vi "SVN Read Disclaimer.vi"(8 "error in (no error)":errorcluster, 9 "Method version":i32, 10 "Method Name":string) -> (0 "error out":errorcluster, 1 "Valid method":bool, 3 "Disclaimer text":string)   [LabVIEW 2012]
uses:
  ReadWrite.ctl
  Folders.ctl
  Design Server.lvlib
panel:
  out "result string":string
  out "standard error":string
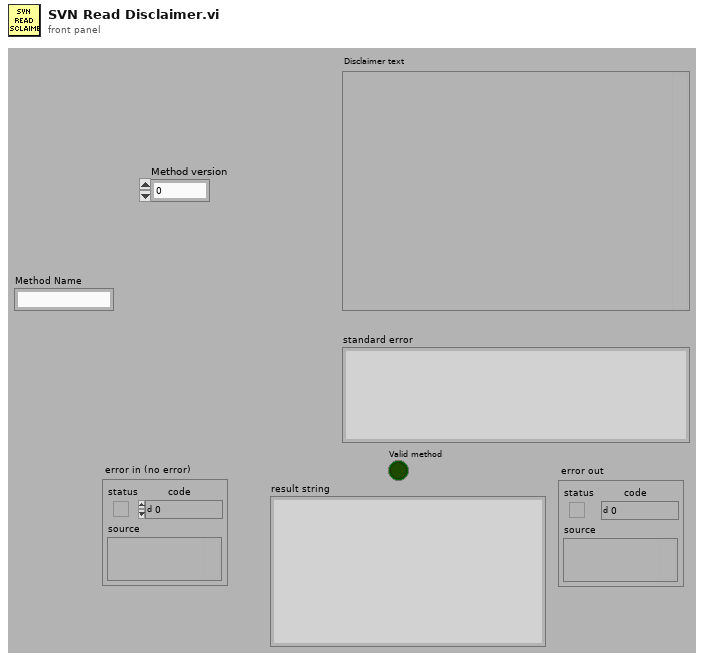
[diagram p1: front panel]
types:
  T1 = typedef "Design Server.lvlib/Folders.ctl" = enum16{"MathcadMethods", "RequestedDesigns", "CompletedDesigns", "MathcadCode", "CollabnetSVN.exe"}
  T2 = typedef "ReadWrite.ctl" = enum16{"Read", "Write"}
  T3 = typedef "SVN.ctl" = cluster{"Mathcad Code Repository":string, "Username":string, "Password":string, "Method file names (w extension)":string}
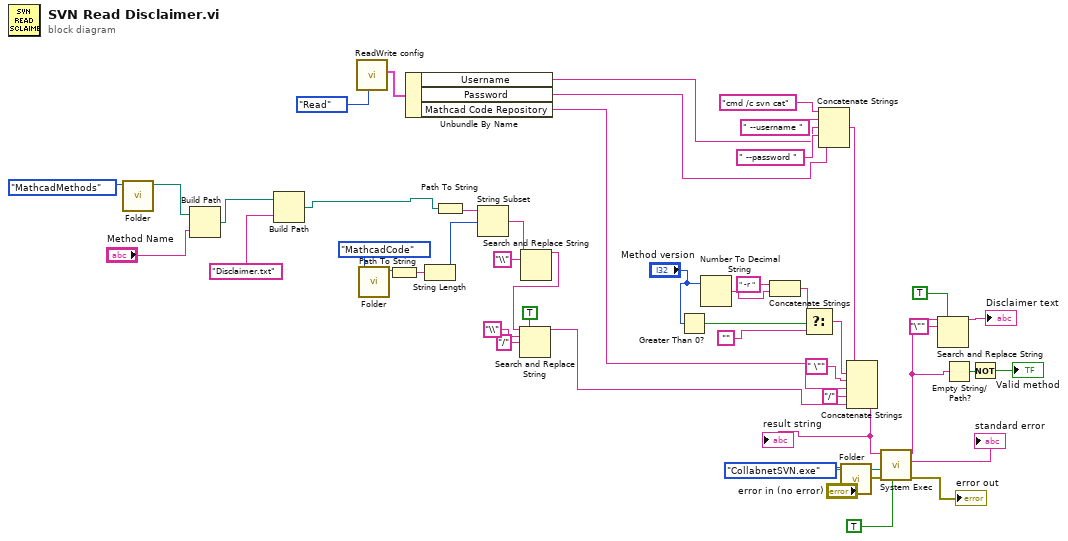
[diagram p0: block diagram]
diagram:
  n1 = call "Folder.vi"("Folders"=Folders."MathcadMethods") -> ("FolderPath"=w4:path)  [unwired: 8 in, 2 out]
  n2 = Build Path(base path=w4, name or relative path="Method Name") -> (appended path=w3:path)
  n3 = Build Path(base path=w3, name or relative path="Disclaimer.txt" ("string")) -> (appended path=w1:path)
  n4 = call "ReadWrite config.vi"("Config"=ReadWrite."Read") -> ("SVN"=w37:T3)  [unwired: 7 in, 3 out]
  n5 = call "Folder.vi"("Folders"=Folders."MathcadCode") -> ("FolderPath"=w25:path)  [unwired: 8 in, 2 out]
  n6 = Path To String(path=w25) -> (string=w26:string)
  n7 = Unbundle By Name(w37) -> ("Username"=w34:string, "Password"=w36:string, "Mathcad Code Repository"=w29:string)
  n8 = String Length(string=w26) -> (length=w22:i32)
  n9 = Path To String(path=w1) -> (string=w2:string)
  n10 = String Subset(string=w2, offset (0)=w22) -> (substring=w21:string)  [unwired: 1 in]
  n11 = Search and Replace String(input string=w21, search string="\\") -> (result string=w18:string)  [unwired: 6 in, 3 out]
  n12 = Search and Replace String(replace all?=TRUE ("replace all? (F)"), input string=w18, search string="\\", replace string="/" ("replace string (\"\")")) -> (result string=w7:string)  [unwired: 4 in, 3 out]
  n13 = Greater Than 0?(x="Method version") -> (x > 0?=w44:bool)
  n14 = Number To Decimal String(number="Method version") -> (decimal integer string=w40:string)  [unwired: 1 in]
  n15 = Concatenate Strings(" -r " ("string"), w40) -> (w42:string)
  n16 = Select(t=w42, s=w44, f="") -> (s? t:f=w39:string)
  n17 = Concatenate Strings("cmd /c svn cat" ("command"), " --username " ("string"), w34, " --password " ("string"), w36) -> (w30:string)
  n18 = call "Folder.vi"("Folders"=Folders."CollabnetSVN.exe") -> ("FolderPath"=w27:path)  [unwired: 8 in, 2 out]
  n19 = Concatenate Strings(w30, w39, " \"" ("string"), w29, "/" ("string"), w7) -> (w6:string)
  "result string" <- w6
  n20 = call <vilib>:"System Exec.vi"("run minimized? (F)"=TRUE, "error in (no error)"="error in (no error)", "working directory"=w27, "command line"=w6) -> ("error out"=→"error out":errorcluster, "standard error"=→"standard error":string, "standard output"=w13:string)  [unwired: 4 in, 1 out]
  n21 = Search and Replace String(replace all?=TRUE ("replace all? (F)"), input string=w13, search string="\"") -> (result string=→"Disclaimer text":string)  [unwired: 5 in, 3 out]
  n22 = Empty String/Path?(string/path=w13) -> (empty?=w15:bool)
  n23 = Not(x=w15) -> (.not. x?=→"Valid method":bool)
